vi "symbol_energy.vi"(9 "Symbol Energy":dbl=1.0 format="%#_4p", 11 "Input Symbols":cdb[](array[numeric])) -> (3 "Output Symbols":cdb[](array[numeric]))   [LabVIEW 2012]
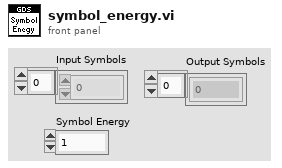
[diagram p1: front panel]
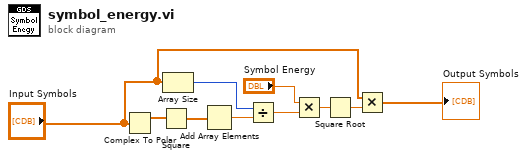
[diagram p0: block diagram]
diagram:
  n1 = Complex To Polar(r * e^(i*theta)="Input Symbols") -> (r=w8:dbl[])  [unwired: 1 out]
  n2 = Square(x=w8) -> (x^2=w7:dbl[])
  n3 = Array Size(array="Input Symbols") -> (size(s)=w9:i32)
  n4 = Add Array Elements(numeric array=w7) -> (sum=w10:dbl)
  n5 = Divide(x=w9, y=w10) -> (x/y=w6:dbl)
  n6 = Multiply(x="Symbol Energy", y=w6) -> (x*y=w5:dbl)
  n7 = Square Root(x=w5) -> (sqrt(x)=w4:dbl)
  n8 = Multiply(x="Input Symbols", y=w4) -> (x*y=→"Output Symbols":cdb[])
